vi "Assert Loopback Value Matches Expected Value.vi"(8 "error in (no error)":errorcluster, 9 "Expected Value":u8, 10 "FPGA VI Reference in":refnum<k20>, 11 "SLSC EDS System Tests in":refnum<class "SLSC EDS System Tests.lvclass">) -> (0 "error out":errorcluster, 2 "FPGA VI Reference Out":refnum<k20>, 3 "SLSC EDS System Tests out":refnum<class "SLSC EDS System Tests.lvclass">)   [LabVIEW 2015, in "SLSC EDS System Tests.lvclass"]
uses:
  SLSC EDS System Tests.lvclass
  <vilib>/Utility/error.llb/Error Cluster From Error Code.vi
  <vilib>/rvi/errors/niLvFpgaAdjustHostInterfaceError.vi
  <vilib>/rvi/interface/nirviReadWriteControl/nirviReadWriteControl.xnode
  NiFpgaLv.dll
  <vilib>/rvi/interface/Simulation/niFpgaSimulationCallBeginRW.vi
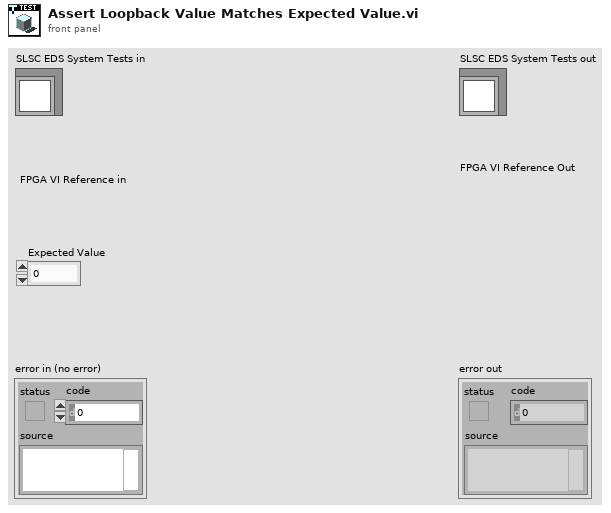
[diagram p1: front panel]
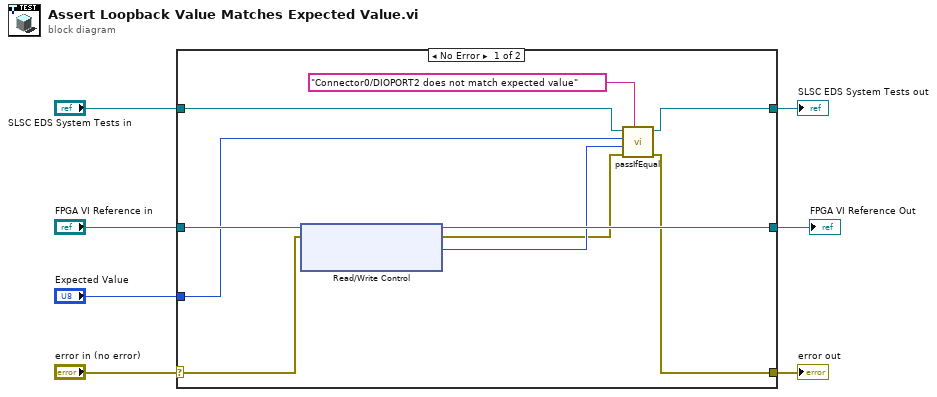
[diagram p0: block diagram]
diagram:
  n1 = case shown="No Error" "error in (no error)" {
    selector: "error in (no error)" -> [w9 w20]
    tunnel: [w11 w20] -> w6
    tunnel: [w14 w19] -> w4
    tunnel: "SLSC EDS System Tests in" -> [w15 w19]
    tunnel: "FPGA VI Reference in" -> [w17 w18]
    tunnel: [w16 w18] -> w2
    tunnel: "Expected Value" -> [w13 _]
    frame No Error {
      n2 = xnode "Read/Write Control"("FPGA VI Reference In"=w17, "error in"=w9) -> ("FPGA VI Reference Out"=w16:refnum<k20>, "error out"=w8:errorcluster, "Connector0/DIOPORT2"=w12:u8)  [unwired: 1 out]
      n3 = call-dynamic "passIfEqual.vi"("custom report message (\"\")"="Connector0/DIOPORT2 does not match expected value" ("custom report message (\"\")"), "error in (no error)"=w8, "y"=w12, "x"=w13, "TestCase in"=w15) -> ("error out"=w11:errorcluster, "TestCase out"=w14:refnum<class "SLSC EDS System Tests.lvclass">)  [unwired: 5 in]
    }
    frame Error {
    }
  }
  "error out" <- w6
  "SLSC EDS System Tests out" <- w4
  "FPGA VI Reference Out" <- w2
